vi "Get Time.vi"() -> (2 "Hora":string, 3 "Fecha":string)   [LabVIEW 2019, in "Base de datos.lvlib"]
uses:
  Documents/Proyecto1/Proyecto1/Libraries/Base de datos/Base de datos.lvlib
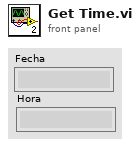
[diagram p1: front panel]
types:
  T1 = typedef "LVDateTimeRec.ctl" = cluster{"fractional second":dbl, "second":i32, "minute":i32, "hour":i32, "day of month":i32, "month":i32, "year":i32, "day of week":i32, "day of year":i32, "DST":i32}
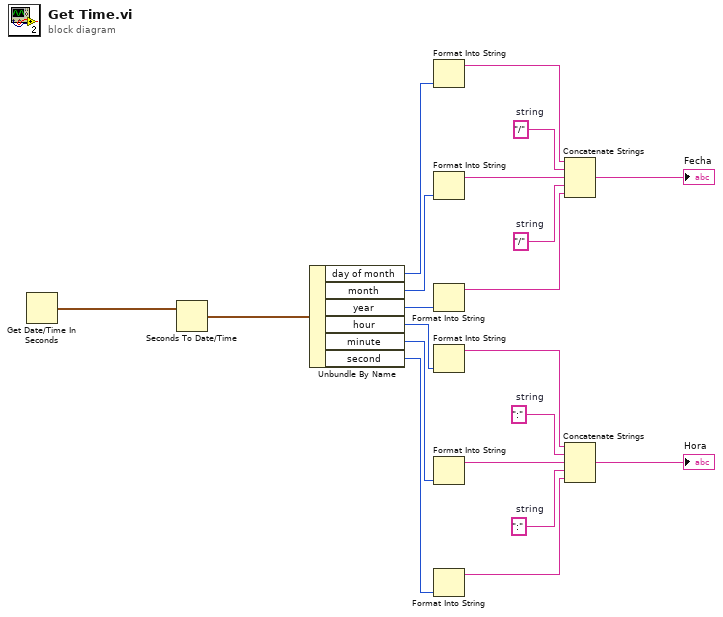
[diagram p0: block diagram]
diagram:
  w1 = ":"  # string
  w5 = ":"  # string
  w9 = "/"  # string
  w10 = "/"  # string
  n1 = Get Date/Time In Seconds() -> (seconds since 1Jan1904=w19:timestamp)
  n2 = Seconds To Date/Time(time stamp (now)=w19) -> (date time rec=w20:T1)  [unwired: 1 in]
  n3 = Unbundle By Name "Unbundle By Name"(w20) -> ("day of month"=w18:i32, "month"=w17:i32, "year"=w16:i32, "hour"=w15:i32, "minute"=w14:i32, "second"=w3:i32)
  n4 = Format Into String "Format Into String"(w18) -> (resulting string=w13:string)  [unwired: 3 in, 1 out]
  n5 = Format Into String "Format Into String"(w17) -> (resulting string=w12:string)  [unwired: 3 in, 1 out]
  n6 = Format Into String "Format Into String"(w16) -> (resulting string=w11:string)  [unwired: 3 in, 1 out]
  n7 = Format Into String "Format Into String"(w15) -> (resulting string=w7:string)  [unwired: 3 in, 1 out]
  n8 = Format Into String "Format Into String"(w14) -> (resulting string=w6:string)  [unwired: 3 in, 1 out]
  n9 = Format Into String "Format Into String"(w3) -> (resulting string=w2:string)  [unwired: 3 in, 1 out]
  n10 = Concatenate Strings "Concatenate Strings"(w13, w10, w12, w9, w11) -> (→"Fecha":string)
  n11 = Concatenate Strings "Concatenate Strings"(w7, w5, w6, w1, w2) -> (→"Hora":string)
